vi "Close Project References.vi"(8 "error in":errorcluster, 11 "Project Refs":refnum<vi>[](array[refnum])) -> (0 "error out":errorcluster)   [LabVIEW 2022 SP3]
doc: "This VI closes any Project references that were open during the execution of the tool.\n\nError behaviour: Execute even if input error"
panel:
  out "Iteration":i32
  # "Development\ncontrols/indicators useful for development and testing, but which are not outputs of the VI"
  # "Input\nInputs to the VI"
  # "Output\nOutputs of the VI"
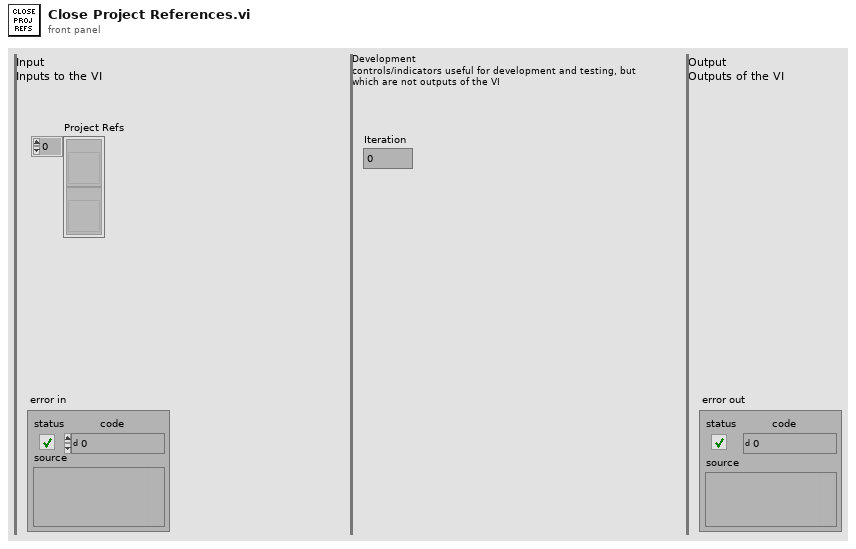
[diagram p1: front panel]
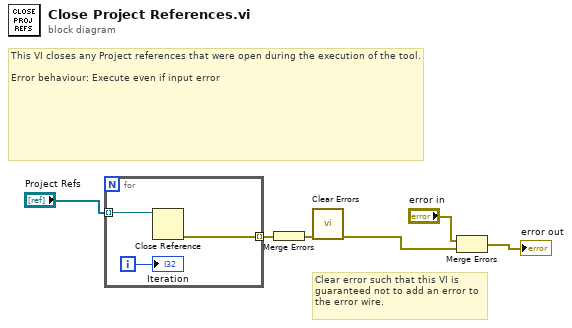
[diagram p0: block diagram]
diagram:
  # "Clear error such that this VI is guaranteed not to add an error to the error wire."
  # "This VI closes any Project references that were open during the execution of the tool.\n\nError behaviour: Execute even if input error"
  n1 = for {
    tunnel: [w9] -> w6 mode=indexing
    tunnel: "Project Refs" -> [w8] mode=indexing
    i -> [w7]
    n2 = Close Reference(reference=w8) -> (error out=w9:errorcluster)  [unwired: 1 in]
    "Iteration" <- w7
  }
  n3 = Merge Errors(w6) -> (w1:errorcluster)
  n4 = call <vilib>:"Clear Errors.vi"("error in (no error)"=w1) -> ("error out"=w2:errorcluster)  [unwired: 5 in, 1 out]
  n5 = Merge Errors("error in", w2) -> (→"error out":errorcluster)
